vi "Find and clear error.vi"(8 "error in (no error)":errorcluster, 10 "error code":i32) -> (0 "error out":errorcluster, 2 "error found?":bool)   [LabVIEW 2023]
doc: "Checks for the given error code and clears it if found."
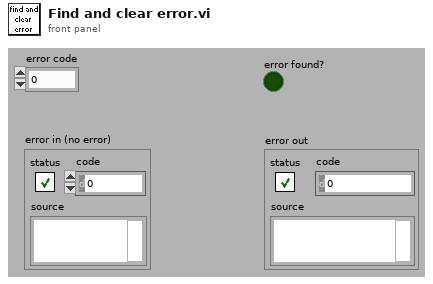
[diagram p1: front panel]
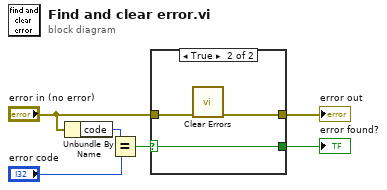
[diagram p0: block diagram]
diagram:
  n1 = Unbundle By Name("error in (no error)") -> ("code"=w5:i32)
  n2 = Equal?(x=w5, y="error code") -> (x = y?=w4:bool)
  n3 = case shown="True" w4 {
    selector: w4 -> [w7 w9]
    tunnel: "error in (no error)" -> [w8 w11]
    tunnel: [w8 w10] -> w1
    tunnel: [w7 w9] -> w2
    frame False {
    }
    frame True {
      n4 = call <vilib>:"Clear Errors.vi"("error in (no error)"=w11) -> ("error out"=w10:errorcluster)  [unwired: 1 in, 5 out]
    }
  }
  "error found?" <- w2
  "error out" <- w1
